vi "Do.vi"(8 "error in":errorcluster, 10 "Actor in":refnum<class "Actor.lvclass">, 11 "Change File Writing State MSG":refnum<class "Change File Writing State MSG.lvclass">) -> (0 "error out":errorcluster, 2 "Actor out":refnum<class "Actor.lvclass">)   [LabVIEW 2014, in "File Library.lvlib" / "Change File Writing State MSG.lvclass"]
doc: "(<B>Filename</B>: Actor Framework.lvlib:Message.lvclass:Do.vi)\n\nDefines what a message does when it is received by an actor. Generally, a message instructs an actor to invoke one of its methods. By default, this method does nothing. A child class must override it to define behavior. Create a child class by using the Actor Framework Message Maker dialog box."
uses:
  Change File Writing State MSG.lvclass
  <vilib>/ActorFramework/Actor/Actor.lvclass
  File Actor.lvclass
  File Actor.lvclass/File Actor.ctl
  Change File Writing State MSG.lvclass/Change File Writing State MSG.ctl
  Read Save DVR.vi
  Read Registration Complete.vi
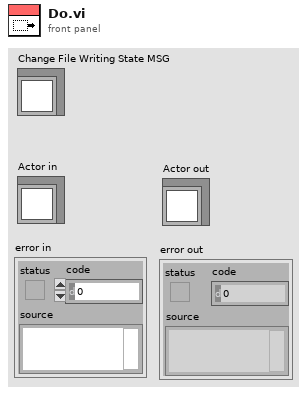
[diagram p1: front panel]
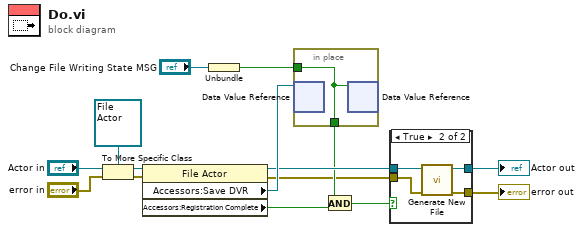
[diagram p0: block diagram]
diagram:
  n1 = To More Specific Class(target class=refnum<class "File Actor.lvclass"> refnum ("File Library.lvlib:File Actor"), reference="Actor in", error in="error in") -> (specific class reference=w11:refnum<class "File Actor.lvclass">, error out=w1:errorcluster)
  n2 = property class="File Actor"(reference=w11, error in=w1) -> (reference out=w8:refnum<class "File Actor.lvclass">, error out=w2:errorcluster, "Accessors:Save DVR"=w10:refnum<data-value>, "Accessors:Registration Complete"=w6:bool)
  n3 = Unbundle("Change File Writing State MSG") -> (w9:bool)
  n4 = in-place {
    in-place-border: w9 -> [w16]
    in-place-border: [w16] -> w7
    n5 = in-place-dvr #1(w10) -> ()  [unwired: 2 out]
    n6 = in-place-dvr #1(w16) -> ()  [unwired: 2 out]
  }
  n7 = And(x=w7, y=w6) -> (x .and. y?=w5:bool)
  n8 = case shown="True" w5 {
    tunnel: w8 -> [w18 w22]
    tunnel: [w18 w21] -> w4
    tunnel: [w17 w20] -> w3
    tunnel: w2 -> [w17 w19]
    frame False {
    }
    frame True {
      n9 = call "Generate New File.vi"("error in"=w19, "File Actor in"=w22) -> ("error out"=w20:errorcluster, "File Actor out"=w21:refnum<class "File Actor.lvclass">)  [unwired: 8 in]
    }
  }
  "error out" <- w3
  "Actor out" <- w4
